vi "Induction Matrix Solver.vi"(0 "Required Storage (FE)":u64, 1 "Required Provider Rate (FE/t)":u64) -> (13 "Provider Rate (kFE/t)":ext, 15 "Provider Rate (FE/t)":u64, 16 "Fits in Max Structure?":bool, 17 "Storage (GFE)":ext, 18 "Min Internal Volume (m³)":u32, 19 "Storage (FE)":u64, 20 "Basic Cells":u64, 21 "Advanced Cells":u64, 22 "Elite Cells":u64, 23 "Ultimate Cells":u64, 24 "Basic Providers":u64, 25 "Advanced Providers":u64, 26 "Elite Providers":u64, 27 "Ultimate Providers":u64)   [LabVIEW 2023]
panel:
  # "Induction Matrix Requirements"
  # "Induction Matrix Population"
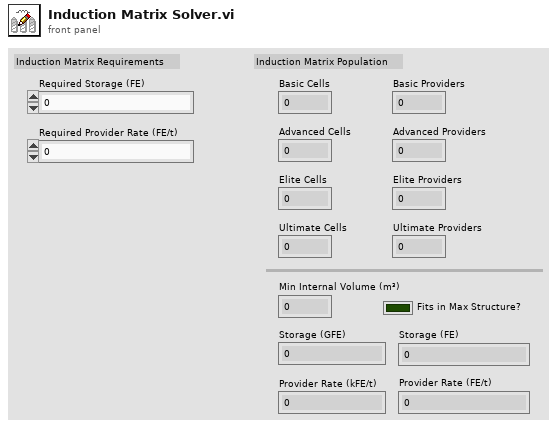
[diagram p1: front panel]
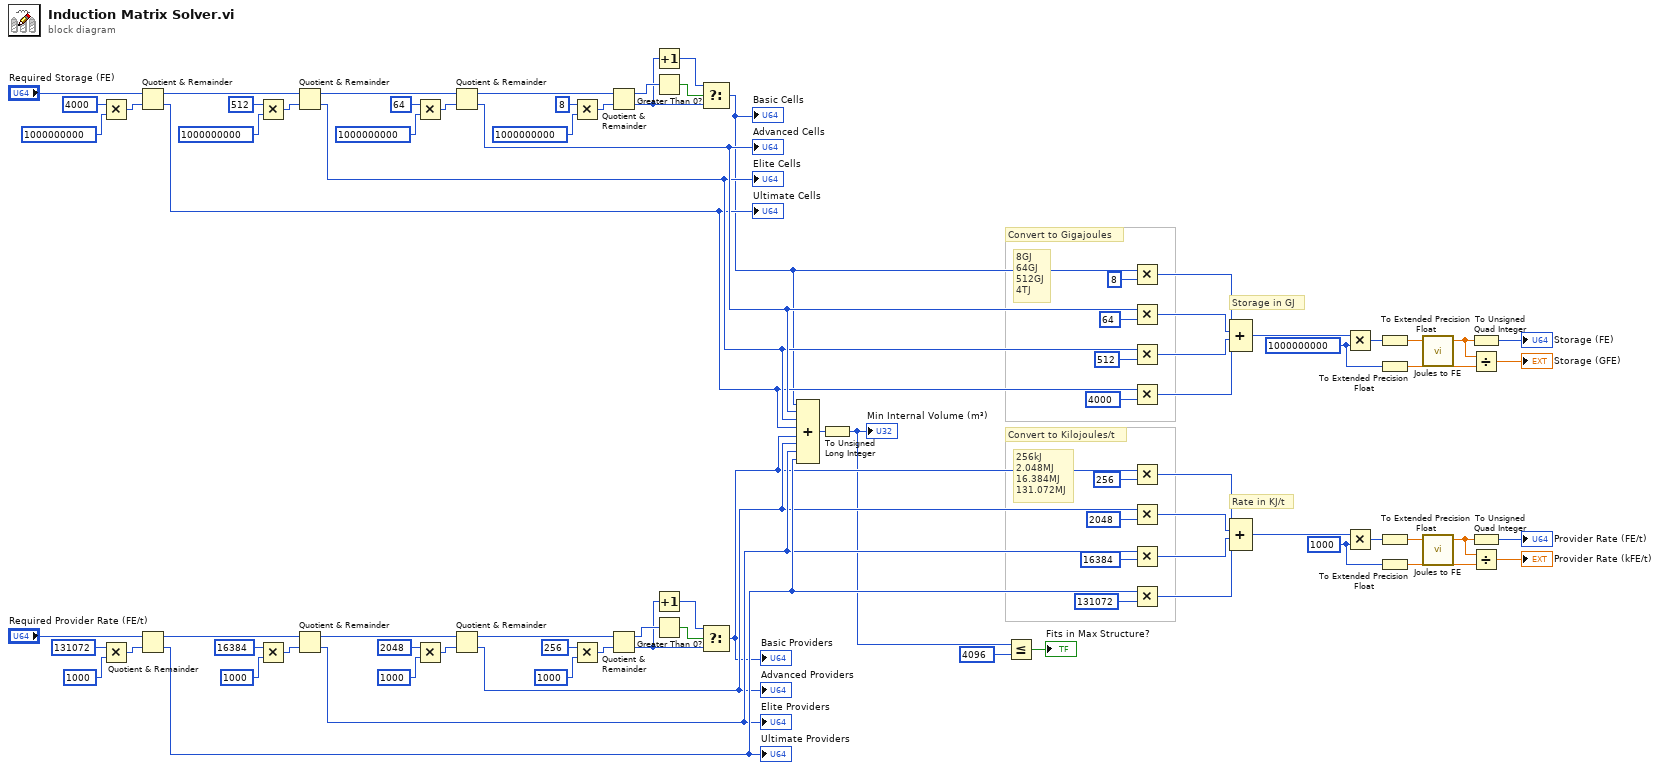
[diagram p0: block diagram]
diagram:
  w59 = u64 1000000000 ("y")
  w62 = u64 1000 ("y")
  # "Rate in KJ/t"
  # "Storage in GJ"
  # "Convert to Kilojoules/t"
  # "256kJ\n2.048MJ\n16.384MJ\n131.072MJ"
  # "8GJ\n64GJ\n512GJ\n4TJ"
  # "Convert to Gigajoules"
  n1 = Multiply(x=u64 4000 ("y"), y=u64 1000000000) -> (x*y=w49:u64)
  n2 = Multiply(x=u64 131072 ("y"), y=u64 1000) -> (x*y=w24:u64)
  n3 = Quotient & Remainder(x="Required Storage (FE)", y=w49) -> (x-y*floor(x/y)=w45:u64, floor(x/y)=w17:u64)
  "Ultimate Cells" <- w17
  n4 = Quotient & Remainder(x="Required Provider Rate (FE/t)", y=w24) -> (x-y*floor(x/y)=w28:u64, floor(x/y)=w16:u64)
  "Ultimate Providers" <- w16
  n5 = Multiply(x=u64 512 ("y"), y=u64 1000000000) -> (x*y=w48:u64)
  n6 = Multiply(x=u64 16384 ("y"), y=u64 1000) -> (x*y=w25:u64)
  n7 = Quotient & Remainder(x=w45, y=w48) -> (x-y*floor(x/y)=w41:u64, floor(x/y)=w18:u64)
  "Elite Cells" <- w18
  n8 = Quotient & Remainder(x=w28, y=w25) -> (x-y*floor(x/y)=w32:u64, floor(x/y)=w15:u64)
  "Elite Providers" <- w15
  n9 = Multiply(x=u64 64 ("y"), y=u64 1000000000) -> (x*y=w42:u64)
  n10 = Multiply(x=u64 2048 ("y"), y=u64 1000) -> (x*y=w31:u64)
  n11 = Quotient & Remainder(x=w41, y=w42) -> (x-y*floor(x/y)=w37:u64, floor(x/y)=w19:u64)
  "Advanced Cells" <- w19
  n12 = Quotient & Remainder(x=w32, y=w31) -> (x-y*floor(x/y)=w36:u64, floor(x/y)=w14:u64)
  "Advanced Providers" <- w14
  n13 = Multiply(x=u64 8 ("y"), y=u64 1000000000) -> (x*y=w40:u64)
  n14 = Multiply(x=u64 256 ("y"), y=u64 1000) -> (x*y=w33:u64)
  n15 = Quotient & Remainder(x=w37, y=w40) -> (x-y*floor(x/y)=w12:u64, floor(x/y)=w9:u64)
  n16 = Quotient & Remainder(x=w36, y=w33) -> (x-y*floor(x/y)=w6:u64, floor(x/y)=w5:u64)
  n17 = Increment(x=w9) -> (x+1=w20:u64)
  n18 = Greater Than 0?(x=w12) -> (x > 0?=w10:bool)
  n19 = Increment(x=w5) -> (x+1=w7:u64)
  n20 = Greater Than 0?(x=w6) -> (x > 0?=w8:bool)
  n21 = Select(t=w20, s=w10, f=w9) -> (s? t:f=w11:u64)
  "Basic Cells" <- w11
  n22 = Select(t=w7, s=w8, f=w5) -> (s? t:f=w4:u64)
  "Basic Providers" <- w4
  n23 = Compound Arithmetic op=ADD(w11, w19, w18, w17, w4, w14, w15, w16) -> (w13:u64)
  n24 = To Unsigned Long Integer(number=w13) -> (unsigned 32bit integer=w2:u32)
  "Min Internal Volume (m³)" <- w2
  n25 = Less Or Equal?(x=w2, y=u32 4096) -> (x <= y?=→"Fits in Max Structure?":bool)
  n26 = Multiply(x=w11, y=u64 8) -> (x*y=w76:u64)
  n27 = Multiply(x=w19, y=u64 64) -> (x*y=w75:u64)
  n28 = Multiply(x=w18, y=u64 512) -> (x*y=w73:u64)
  n29 = Multiply(x=w17, y=u64 4000) -> (x*y=w74:u64)
  n30 = Multiply(x=w4, y=u64 256) -> (x*y=w72:u64)
  n31 = Multiply(x=w14, y=u64 2048) -> (x*y=w71:u64)
  n32 = Multiply(x=w15, y=u64 16384) -> (x*y=w70:u64)
  n33 = Multiply(x=w16, y=u64 131072) -> (x*y=w69:u64)
  n34 = Compound Arithmetic op=ADD(w76, w75, w73, w74) -> (w66:u64)
  n35 = Compound Arithmetic op=ADD(w72, w71, w70, w69) -> (w68:u64)
  n36 = Multiply(x=w66, y=w59) -> (x*y=w65:u64)
  n37 = Multiply(x=w68, y=w62) -> (x*y=w67:u64)
  n38 = To Extended Precision Float(1:w65) -> (0:w64:ext)
  n39 = To Extended Precision Float(1:w59) -> (0:w60:ext)
  n40 = To Extended Precision Float(1:w67) -> (0:w63:ext)
  n41 = To Extended Precision Float(1:w62) -> (0:w61:ext)
  n42 = call "Joules to FE.vi"("J"=w64) -> ("FE"=w56:dbl)  [unwired: 4 in]
  n43 = call "Joules to FE.vi"("J"=w63) -> ("FE"=w54:dbl)  [unwired: 4 in]
  n44 = To Unsigned Quad Integer(1:w56) -> (0:→"Storage (FE)":u64)
  n45 = Divide(x=w56, y=w60) -> (x/y=→"Storage (GFE)":ext)
  n46 = To Unsigned Quad Integer(1:w54) -> (0:→"Provider Rate (FE/t)":u64)
  n47 = Divide(x=w54, y=w61) -> (x/y=→"Provider Rate (kFE/t)":ext)
